vi "Main-top_feature - txtPath.vi"() -> ()   [LabVIEW 2015]
uses:
  <vilib>/Utility/file.llb/Read Delimited Spreadsheet (string).vi
  <vilib>/Utility/file.llb/Write Delimited Spreadsheet (string).vi
  <vilib>/vision/NI_Vision_Development_Module.lvlib
  EG.dll
  greenDet.dll
panel:
  out "Flower":T1(plugin-control)
  out "element":string
  in  "Date Path":path=path "H:/2-top_features_oilseed/date -whole.txt"
  in  "Save Base Path":path=path "H:/2-top_features_oilseed"
  out "交集图":T1(plugin-control)
  out "交集像素个数":dbl
  in  "Pixel Measurements 2":T2[](array[typedef])=[35] items=["Center of Mass X", "Center of Mass Y", "First Pixel X", "First Pixel Y", "Bounding Rect Left", "Bounding Rect Top", "Bounding Rect Right", "Bounding Rect Bottom", "Max Feret Diameter Start X", "Max Feret Diameter Start Y", "Max Feret Diameter End X", "Max Feret Diameter End Y", "Max Horiz. Segment Length Left", "Max Horiz. Segment Length Right", "Max Horiz. Segment Length Row", "-", "Bounding Rect Width", "Bounding Rect Height", "Bounding Rect Diagonal", "Perimeter", "Convex Hull Perimeter", "Holes' Perimeter", "Max Feret Diameter", "Equivalent Ellipse Major Axis", "Equivalent Ellipse Minor Axis", "Equivalent Ellipse Minor Axis (Feret)", "Equivalent Rect Long Side", "Equivalent Rect Short Side", "Equivalent Rect Diagonal", "Equivalent Rect Short Side (Feret)", "Average Horiz. Segment Length", "Average Vert. Segment Length", "Hydraulic Radius", "Waddel Disk Diameter", "-", "Area", "Holes' Area", "Particle & Holes' Area", "Convex Hull Area", "Image Area", "-", "Number of Holes", "Number of Horiz. Segments", "Number of Vert. Segments", "-", "Orientation", "Max Feret Diameter Orientation", "-", "% Area/Image Area", "% Area/(Particle & Holes' Area)", "Ratio of Equivalent Ellipse Axes", "Ratio of Equivalent Rect Sides", "-", "Elongation Factor", "Compactness Factor", "Heywood Circularity Factor", "Type Factor", "-", "Sum X", "Sum Y", "Sum XX", "Sum XY", "Sum YY", "Sum XXX", "Sum XXY", "Sum XYY", "Sum YYY", "-", "Moment of Inertia XX", "Moment of Inertia XY", "Moment of Inertia YY", "Moment of Inertia XXX", "Moment of Inertia XXY", "Moment of Inertia XYY", "Moment of Inertia YYY", "Norm. Moment of Inertia XX", "Norm. Moment of Inertia XY", "Norm. Moment of Inertia YY", "Norm. Moment of Inertia XXX", "Norm. Moment of Inertia XXY", "Norm. Moment of Inertia XYY", "Norm. Moment of Inertia YYY", "Hu Moment 1", "Hu Moment 2", "Hu Moment 3", "Hu Moment 4", "Hu Moment 5", "Hu Moment 6", "Hu Moment 7"]
  in  "Pixel Measurements":T2[](array[typedef])=[35] items=["Center of Mass X", "Center of Mass Y", "First Pixel X", "First Pixel Y", "Bounding Rect Left", "Bounding Rect Top", "Bounding Rect Right", "Bounding Rect Bottom", "Max Feret Diameter Start X", "Max Feret Diameter Start Y", "Max Feret Diameter End X", "Max Feret Diameter End Y", "Max Horiz. Segment Length Left", "Max Horiz. Segment Length Right", "Max Horiz. Segment Length Row", "-", "Bounding Rect Width", "Bounding Rect Height", "Bounding Rect Diagonal", "Perimeter", "Convex Hull Perimeter", "Holes' Perimeter", "Max Feret Diameter", "Equivalent Ellipse Major Axis", "Equivalent Ellipse Minor Axis", "Equivalent Ellipse Minor Axis (Feret)", "Equivalent Rect Long Side", "Equivalent Rect Short Side", "Equivalent Rect Diagonal", "Equivalent Rect Short Side (Feret)", "Average Horiz. Segment Length", "Average Vert. Segment Length", "Hydraulic Radius", "Waddel Disk Diameter", "-", "Area", "Holes' Area", "Particle & Holes' Area", "Convex Hull Area", "Image Area", "-", "Number of Holes", "Number of Horiz. Segments", "Number of Vert. Segments", "-", "Orientation", "Max Feret Diameter Orientation", "-", "% Area/Image Area", "% Area/(Particle & Holes' Area)", "Ratio of Equivalent Ellipse Axes", "Ratio of Equivalent Rect Sides", "-", "Elongation Factor", "Compactness Factor", "Heywood Circularity Factor", "Type Factor", "-", "Sum X", "Sum Y", "Sum XX", "Sum XY", "Sum YY", "Sum XXX", "Sum XXY", "Sum XYY", "Sum YYY", "-", "Moment of Inertia XX", "Moment of Inertia XY", "Moment of Inertia YY", "Moment of Inertia XXX", "Moment of Inertia XXY", "Moment of Inertia XYY", "Moment of Inertia YYY", "Norm. Moment of Inertia XX", "Norm. Moment of Inertia XY", "Norm. Moment of Inertia YY", "Norm. Moment of Inertia XXX", "Norm. Moment of Inertia XXY", "Norm. Moment of Inertia XYY", "Norm. Moment of Inertia YYY", "Hu Moment 1", "Hu Moment 2", "Hu Moment 3", "Hu Moment 4", "Hu Moment 5", "Hu Moment 6", "Hu Moment 7"]
  out "黄色分量（油菜花）二值图":T1(plugin-control)
  out "黄色分量（油菜花）":T1(plugin-control)
  out "Original Image":T1(plugin-control)
  out "Current Path":path
  out "Current Number":string
  in  "ROI_whole":T3={"Top"=550, "im_height"=1000, "L_left"=650, "im_width"=1050}
  in  "Crop image ?":bool
  out "HistStat_whole":dbl[](array[numeric])
  out "AC (Area Convexity)":dbl
  out "P":dbl
  out "TPA (Total projective area)":dbl
  out "SFD":sgl
  out "BW (minimum circumscribed box width)":dbl
  out "BH":dbl
  out "R (Rectangularity)":dbl
  out "IFD":sgl
  out "Hull area":dbl
  out "HWR":dbl
  out "greenDet":dbl
  out "Crop Image":T1(plugin-control)
  out "Final Binary Image":T1(plugin-control)
  in  "EG threshold":sgl=0.15
  in  "ER threshold":sgl=0.6
  out "Final image":T1(plugin-control)
  out "Preliminary image":T1(plugin-control)
  out "GPA (Green projective area)":dbl
  out "YPA (Yellow projective area)":dbl
  out "Image Path":path
  # "Digital evaluation software for oilseed rape phenotype-related traits (top-view) v1.0"
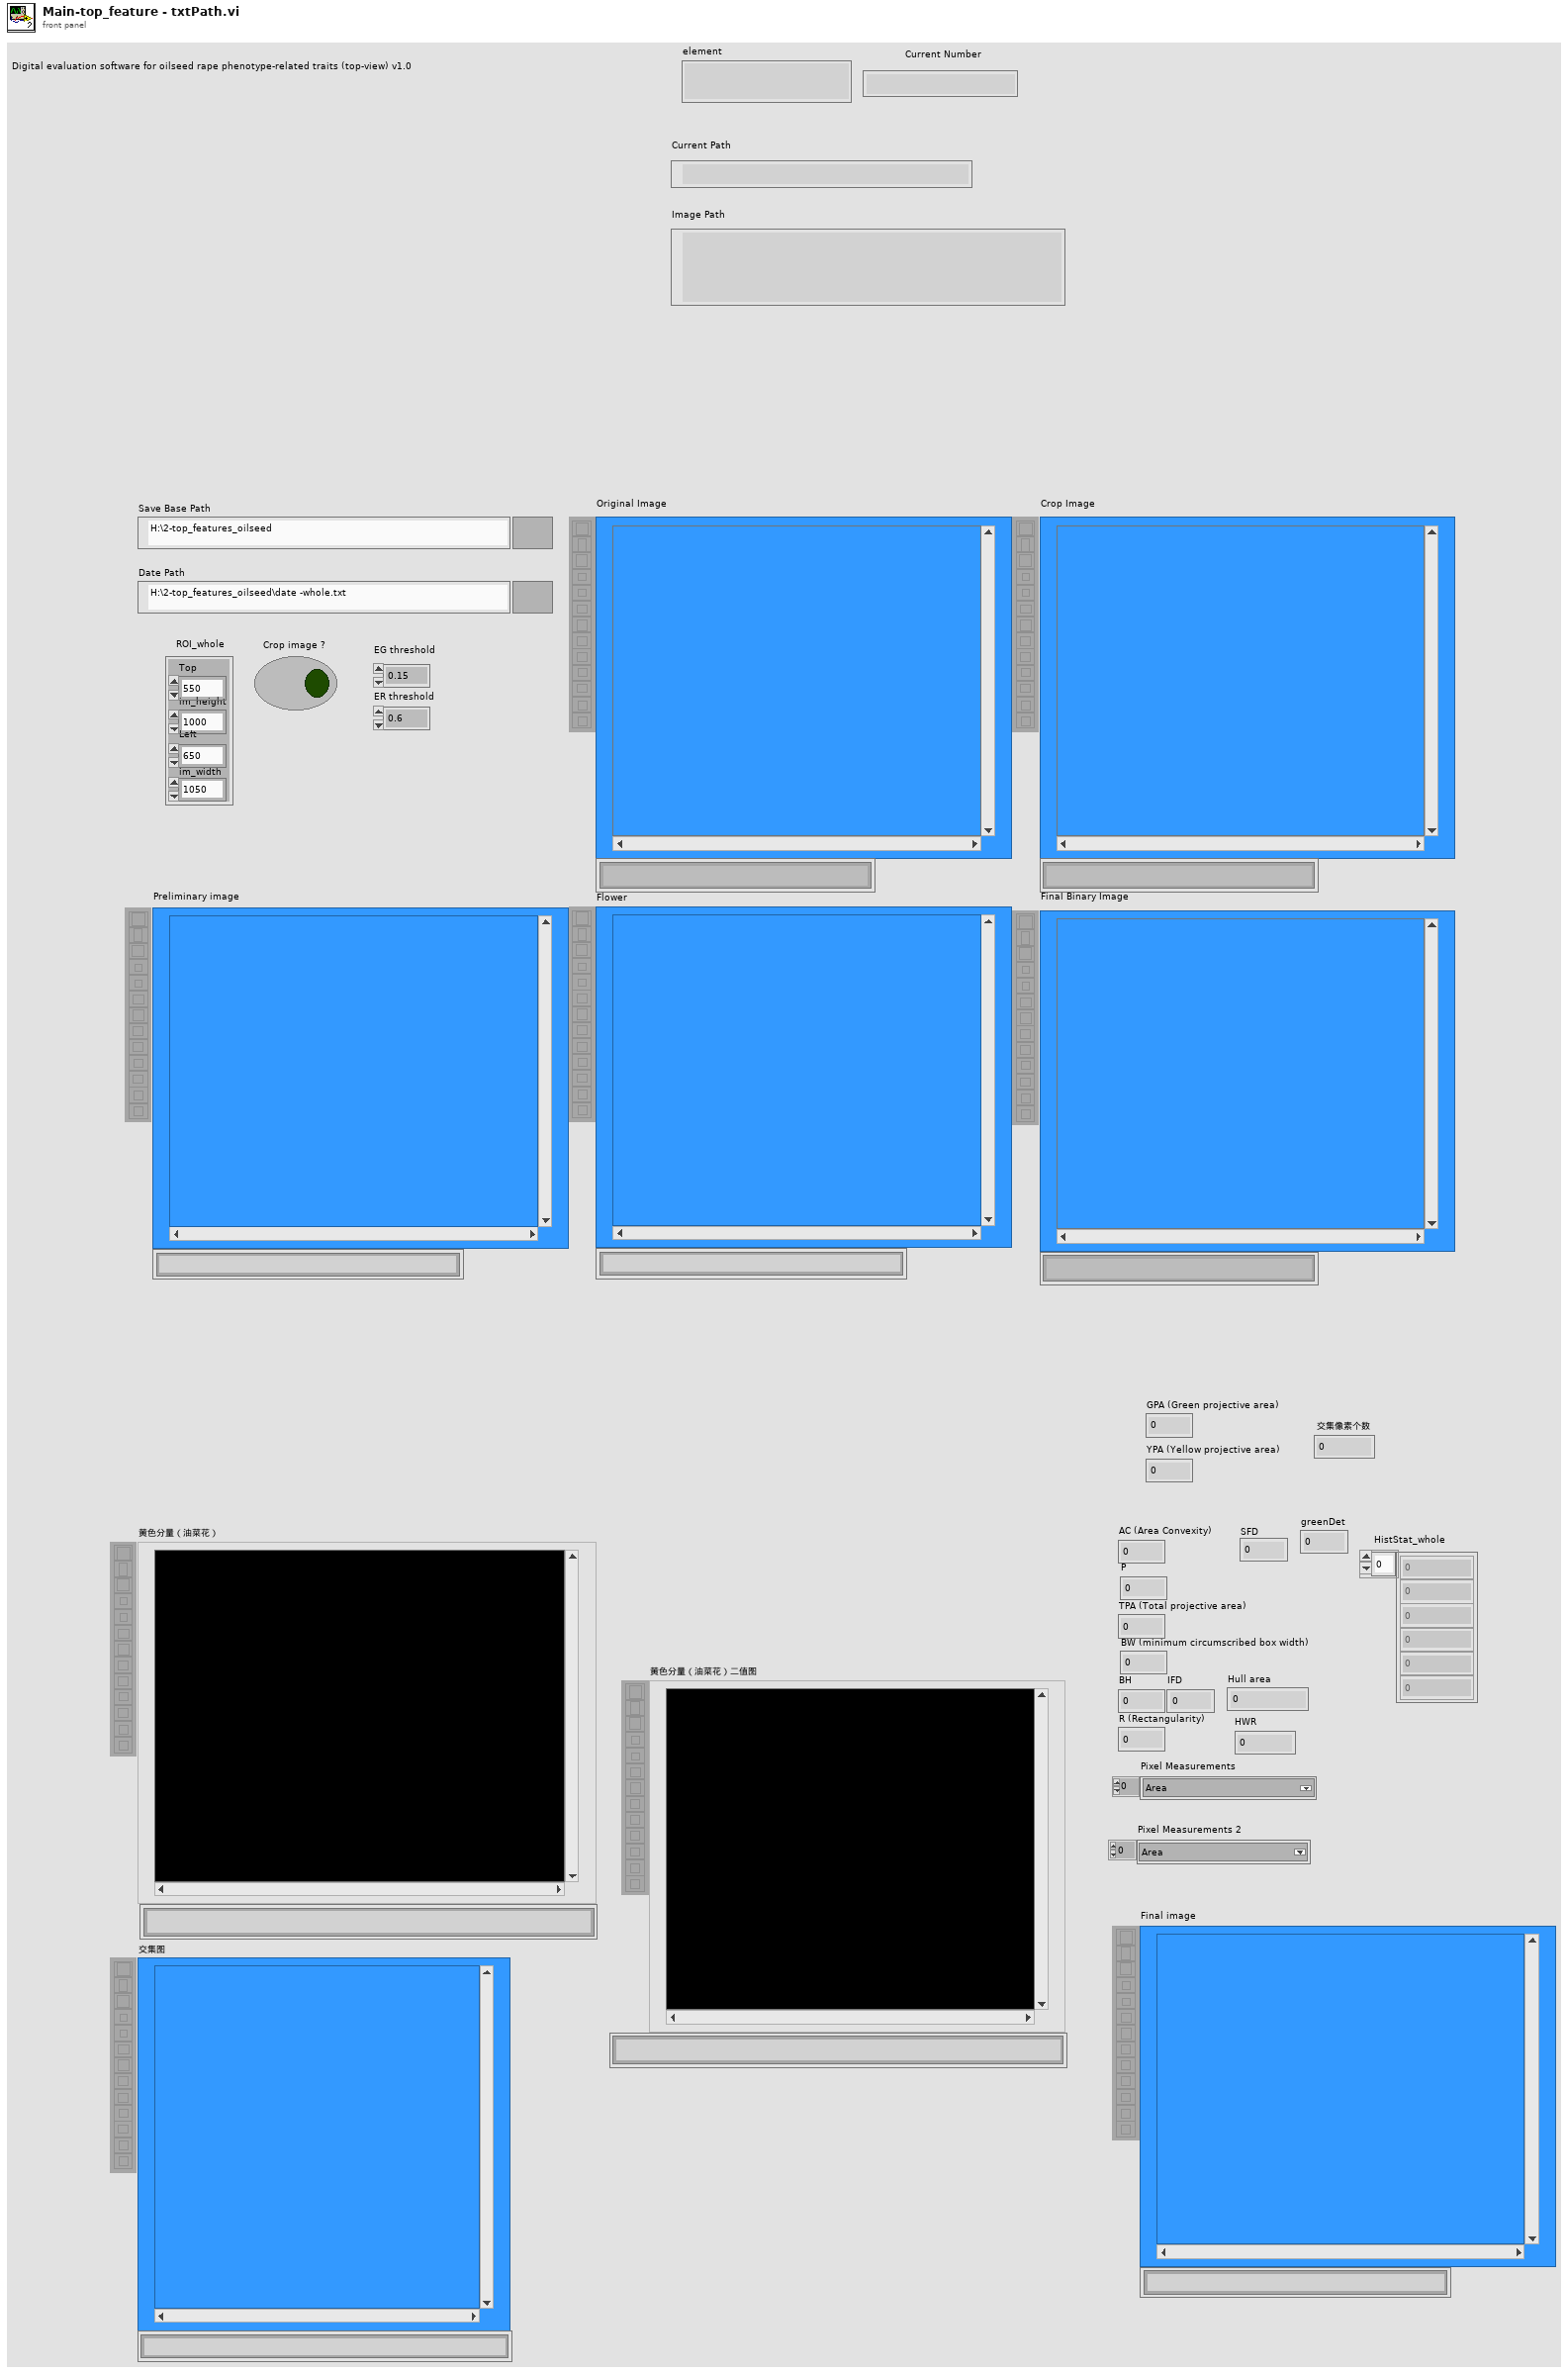
[diagram p1: front panel]
types:
  T1 = typedef "IMAQ Image.ctl" = refnum<image>
  T2 = typedef "Particle Parameters" = i32
  T3 = cluster{"Top":i32, "im_height":i32, "L_left":i32, "im_width":i32}
  T4 = enum32{"AutoM", "Close", "Dilate", "Erode", "Gradient", "Gradient out", "Gradient in", "Hit miss", "Open", "PClose", "POpen", "Thick", "Thin"}
  T5 = typedef "Image Type" = u32
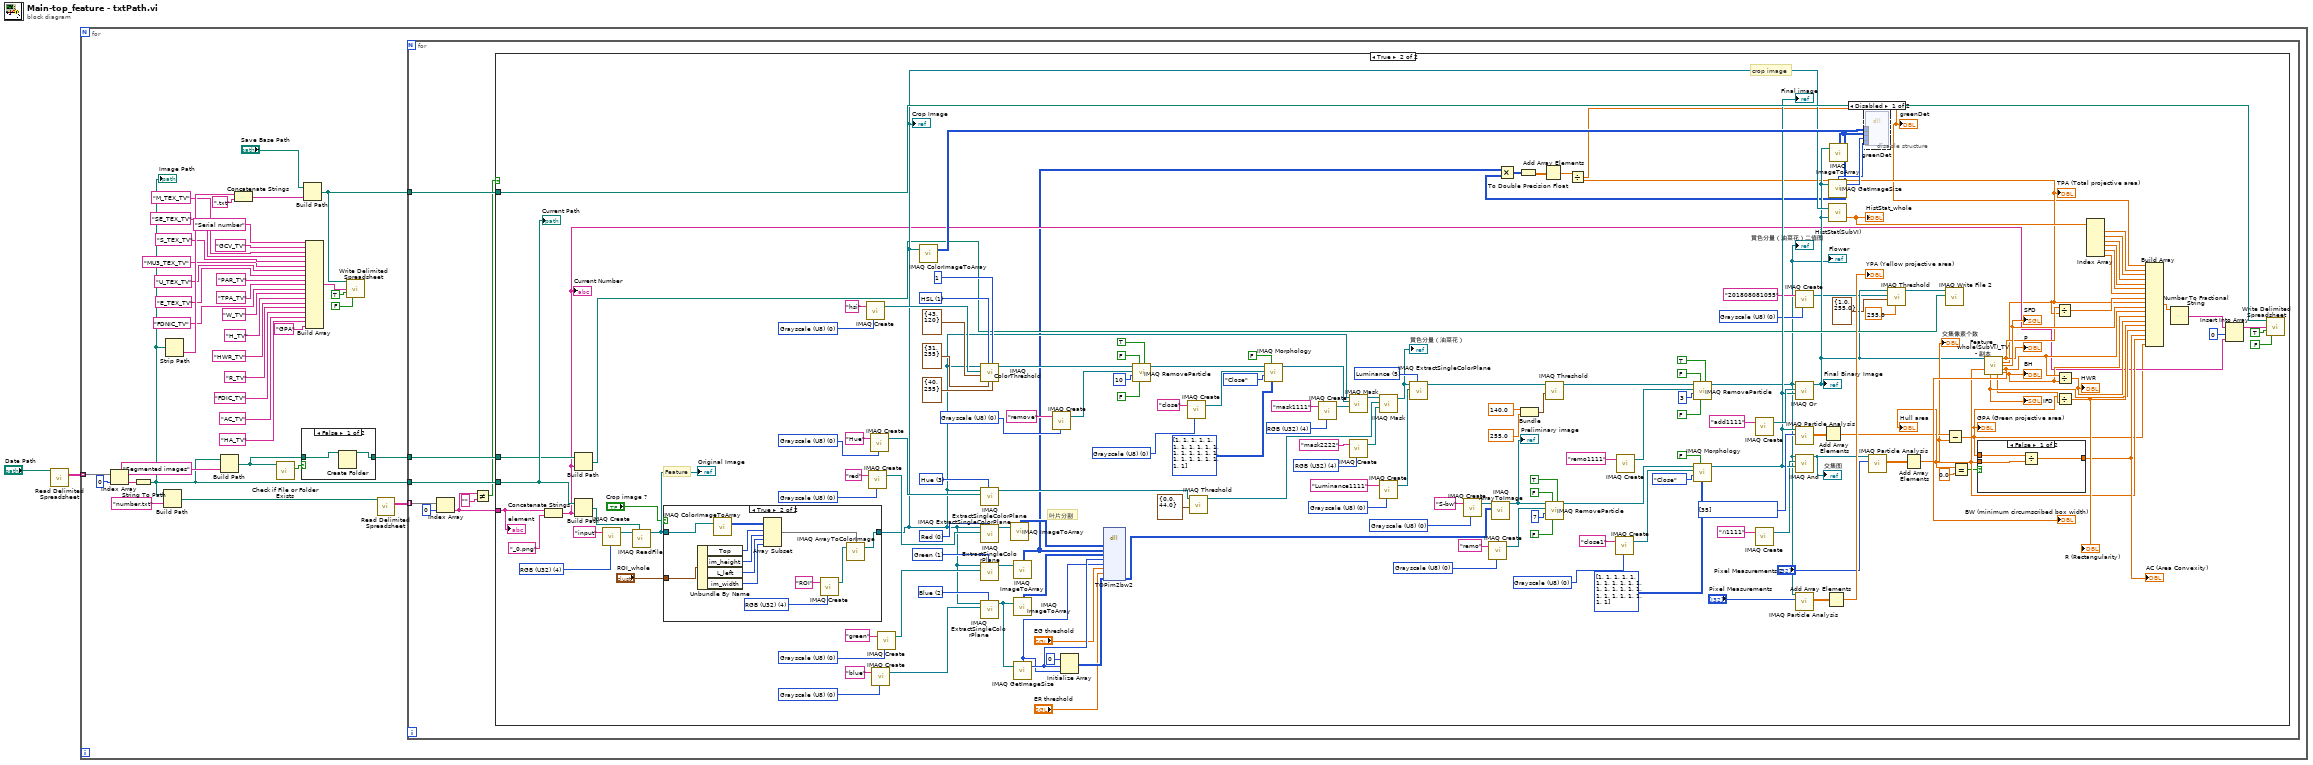
[diagram p0: block diagram]
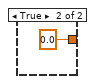
[diagram p5: hidden frame]
diagram:
  n1 = call-poly <vilib>:"Read Delimited Spreadsheet.vi"("file path (dialog if empty)"="Date Path") -> ("all rows"=w1:string[][])  [unwired: 9 in, 5 out]
  n2 = for {
    tunnel: w1 -> [w39] mode=indexing
    n3 = Index Array(array=w39, index=0) -> (element=w28:string)
    n4 = String To Path(string=w28) -> (path=w26:path)
    "Image Path" <- w26
    n5 = Build Path(base path=w26, name or relative path="number.txt") -> (appended path=w37:path)
    n6 = Strip Path(path=w26) -> (name=w27:string)  [unwired: 1 out]
    n7 = Build Path(base path=w26, name or relative path="Segmented images") -> (appended path=w33:path)
    n8 = Concatenate Strings(w27, ".txt" ("string")) -> (w30:string)
    n9 = call <vilib>:"Check if File or Folder Exists.vi"("path"=w33) -> ("file or folder exists?"=w34:bool)  [unwired: 8 in, 2 out]
    n10 = case shown="False" w34 {
      tunnel: [w41 w43] -> w32
      tunnel: w33 -> [w42 w43]
      frame False {
        n11 = Create Folder(path (use dialog)=w42) -> (created path=w41:path)  [unwired: 2 in, 2 out]
      }
      frame True {
      }
    }
    n12 = Build Path(base path="Save Base Path", name or relative path=w30) -> (appended path=w23:path)
    n13 = Build Array("Serial number" ("name or relative path"), "GCV_TV" ("name or relative path"), "M_TEX_TV" ("name or relative path"), "SE_TEX_TV" ("name or relative path"), "S_TEX_TV" ("name or relative path"), "MU3_TEX_TV" ("name or relative path"), "U_TEX_TV" ("name or relative path"), "E_TEX_TV" ("name or relative path"), "PAR_TV" ("name or relative path"), "TPA_TV" ("name or relative path"), "FDNIC_TV" ("name or relative path"), "W_TV" ("name or relative path"), "H_TV" ("name or relative path"), "HWR_TV" ("name or relative path"), "R_TV" ("name or relative path"), "FDIC_TV" ("name or relative path"), "AC_TV" ("name or relative path"), "HA_TV" ("name or relative path"), "GPA" ("name or relative path")) -> (w3:string[])
    n14 = call-poly <vilib>:"Write Delimited Spreadsheet.vi"("file path (dialog if empty)"=w23, "1D data"=w3, "append to file? (F)"=TRUE, "transpose? (F)"=FALSE ("append to file? (new file:F)")) -> ()  [unwired: 10 in, 2 out]
    n15 = call-poly <vilib>:"Read Delimited Spreadsheet.vi"("file path (dialog if empty)"=w37) -> ("all rows"=w36:string[][])  [unwired: 9 in, 5 out]
    n16 = for {
      tunnel: w26 -> [w49]
      tunnel: w36 -> [w50] mode=indexing
      tunnel: w32 -> [w48]
      tunnel: w23 -> [w47]
      n17 = Index Array(array=w50, index=0) -> (element=w46:string)
      n18 = Not Equal?(x=w46, y="") -> (x != y?=w44:bool)
      n19 = case shown="True" w44 {
        tunnel: w49 -> [_ w222]
        tunnel: w48 -> [_ w203]
        tunnel: w47 -> [_ w202]
        tunnel: w46 -> [_ w63]
        frame False {
        }
        frame True {
          w73 = u32 0 items=["Grayscale (U8)", "Grayscale (I16)", "Grayscale (SGL)", "Complex (CSG)", "RGB (U32)", "HSL (U32)", "RGB (U64)"] ("Image Type")
          w102 = u32 0 items=["Grayscale (U8)", "Grayscale (I16)", "Grayscale (SGL)", "Complex (CSG)", "RGB (U32)", "HSL (U32)", "RGB (U64)"] ("Image Type")
          w105 = 5 items=["Red", "Green", "Blue", "Hue", "Saturation", "Luminance", "Value", "Intensity"] ("Color Plane")
          w109 = u32 0 items=["Grayscale (U8)", "Grayscale (I16)", "Grayscale (SGL)", "Complex (CSG)", "RGB (U32)", "HSL (U32)", "RGB (U64)"] ("Image Type")
          w112 = 3 items=["Red", "Green", "Blue", "Hue", "Saturation", "Luminance", "Value", "Intensity"] ("Color Plane")
          w115 = u32 4 items=["Grayscale (U8)", "Grayscale (I16)", "Grayscale (SGL)", "Complex (CSG)", "RGB (U32)", "HSL (U32)", "RGB (U64)"] ("Image Type")
          w118 = u32 4 items=["Grayscale (U8)", "Grayscale (I16)", "Grayscale (SGL)", "Complex (CSG)", "RGB (U32)", "HSL (U32)", "RGB (U64)"] ("Image Type")
          w127 = u32 0 items=["Grayscale (U8)", "Grayscale (I16)", "Grayscale (SGL)", "Complex (CSG)", "RGB (U32)", "HSL (U32)", "RGB (U64)"] ("Image Type")
          w131 = T2[] [35] items=["Center of Mass X", "Center of Mass Y", "First Pixel X", "First Pixel Y", "Bounding Rect Left", "Bounding Rect Top", "Bounding Rect Right", "Bounding Rect Bottom", "Max Feret Diameter Start X", "Max Feret Diameter Start Y", "Max Feret Diameter End X", "Max Feret Diameter End Y", "Max Horiz. Segment Length Left", "Max Horiz. Segment Length Right", "Max Horiz. Segment Length Row", "-", "Bounding Rect Width", "Bounding Rect Height", "Bounding Rect Diagonal", "Perimeter", "Convex Hull Perimeter", "Holes' Perimeter", "Max Feret Diameter", "Equivalent Ellipse Major Axis", "Equivalent Ellipse Minor Axis", "Equivalent Ellipse Minor Axis (Feret)", "Equivalent Rect Long Side", "Equivalent Rect Short Side", "Equivalent Rect Diagonal", "Equivalent Rect Short Side (Feret)", "Average Horiz. Segment Length", "Average Vert. Segment Length", "Hydraulic Radius", "Waddel Disk Diameter", "-", "Area", "Holes' Area", "Particle & Holes' Area", "Convex Hull Area", "Image Area", "-", "Number of Holes", "Number of Horiz. Segments", "Number of Vert. Segments", "-", "Orientation", "Max Feret Diameter Orientation", "-", "% Area/Image Area", "% Area/(Particle & Holes' Area)", "Ratio of Equivalent Ellipse Axes", "Ratio of Equivalent Rect Sides", "-", "Elongation Factor", "Compactness Factor", "Heywood Circularity Factor", "Type Factor", "-", "Sum X", "Sum Y", "Sum XX", "Sum XY", "Sum YY", "Sum XXX", "Sum XXY", "Sum XYY", "Sum YYY", "-", "Moment of Inertia XX", "Moment of Inertia XY", "Moment of Inertia YY", "Moment of Inertia XXX", "Moment of Inertia XXY", "Moment of Inertia XYY", "Moment of Inertia YYY", "Norm. Moment of Inertia XX", "Norm. Moment of Inertia XY", "Norm. Moment of Inertia YY", "Norm. Moment of Inertia XXX", "Norm. Moment of Inertia XXY", "Norm. Moment of Inertia XYY", "Norm. Moment of Inertia YYY", "Hu Moment 1", "Hu Moment 2", "Hu Moment 3", "Hu Moment 4", "Hu Moment 5", "Hu Moment 6", "Hu Moment 7"] ("Pixel Measurements")
          w164 = T5 0 items=["Grayscale (U8)", "Grayscale (I16)", "Grayscale (SGL)", "Complex (CSG)", "RGB (U32)", "HSL (U32)", "RGB (U64)", "Grayscale (U16)"] ("Image Type")
          w157 = T5 0 items=["Grayscale (U8)", "Grayscale (I16)", "Grayscale (SGL)", "Complex (CSG)", "RGB (U32)", "HSL (U32)", "RGB (U64)", "Grayscale (U16)"] ("Image Type")
          w144 = 2 items=["Red", "Green", "Blue", "Hue", "Saturation", "Luminance", "Value", "Intensity"] ("Color Plane")
          w143 = 0 items=["Red", "Green", "Blue", "Hue", "Saturation", "Luminance", "Value", "Intensity"] ("Color Plane")
          w140 = T5 0 items=["Grayscale (U8)", "Grayscale (I16)", "Grayscale (SGL)", "Complex (CSG)", "RGB (U32)", "HSL (U32)", "RGB (U64)", "Grayscale (U16)"] ("Image Type")
          w138 = 1 items=["Red", "Green", "Blue", "Hue", "Saturation", "Luminance", "Value", "Intensity"] ("Color Plane")
          w135 = T5 0 items=["Grayscale (U8)", "Grayscale (I16)", "Grayscale (SGL)", "Complex (CSG)", "RGB (U32)", "HSL (U32)", "RGB (U64)", "Grayscale (U16)"] ("Image Type")
          w139 = T5 0 items=["Grayscale (U8)", "Grayscale (I16)", "Grayscale (SGL)", "Complex (CSG)", "RGB (U32)", "HSL (U32)", "RGB (U64)", "Grayscale (U16)"] ("Image Type")
          w168 = u32 0 items=["Grayscale (U8)", "Grayscale (I16)", "Grayscale (SGL)", "Complex (CSG)", "RGB (U32)", "HSL (U32)", "RGB (U64)"] ("Image Type")
          w179 = u32 0 items=["Grayscale (U8)", "Grayscale (I16)", "Grayscale (SGL)", "Complex (CSG)", "RGB (U32)", "HSL (U32)", "RGB (U64)"] ("Image Type")
          w182 = u32 0 items=["Grayscale (U8)", "Grayscale (I16)", "Grayscale (SGL)", "Complex (CSG)", "RGB (U32)", "HSL (U32)", "RGB (U64)"] ("Image Type")
          w184 = u16 1 items=["RGB", "HSL", "HSV", "HSI"] ("Color Mode")
          w199 = T5 4 items=["Grayscale (U8)", "Grayscale (I16)", "Grayscale (SGL)", "Complex (CSG)", "RGB (U32)", "HSL (U32)", "RGB (U64)", "Grayscale (U16)"] ("Image Type")
          # "叶片分割"
          # "crop image"
          # "Feature"
          n20 = Concatenate Strings(w63, "_0.png" ("string")) -> (w61:string)
          "Current Number" <- w61
          n21 = Build Path(base path=w203, name or relative path=w61) -> (appended path=w75:path)
          n22 = Build Path(base path=w222, name or relative path=w61) -> (appended path=w198:path)
          n23 = call "IMAQ Create"("Image Name"="input", "Image Type"=w199) -> ("New Image"=w200:T1)  [unwired: 2 in, 2 out]
          n24 = call "IMAQ ReadFile"("File Path"=w198, "Image"=w200) -> ("Image Out"=w196:T1)  [unwired: 3 in, 6 out]
          "Original Image" <- w196
          n25 = case shown="True" "Crop image ?" {
            tunnel: w196 -> [w231 w238]
            tunnel: "ROI_whole" -> [_ w233]
            tunnel: [w231 w232] -> w87
            frame False {
            }
            frame True {
              w236 = u32 4 items=["Grayscale (U8)", "Grayscale (I16)", "Grayscale (SGL)", "Complex (CSG)", "RGB (U32)", "HSL (U32)", "RGB (U64)"] ("Image Type")
              n26 = Unbundle By Name(w233) -> ("Top"=w240:i32, "im_height"=w241:i32, "L_left"=w242:i32, "im_width"=w243:i32)
              n27 = call "IMAQ ColorImageToArray"("Image"=w238) -> ("Image Pixels (U32)"=w239:u32[][])  [unwired: 2 in, 3 out]
              n28 = Array Subset(array=w239, index (row)=w240, length (row)=w241, index (col)=w242, length (col)=w243) -> (w234:u32[][])
              n29 = call "IMAQ Create"("Image Name"="ROI", "Image Type"=w236) -> ("New Image"=w235:T1)  [unwired: 2 in, 2 out]
              n30 = call "IMAQ ArrayToColorImage"("Image Pixels (U32)"=w234, "Image"=w235) -> ("Image Out"=w232:T1)  [unwired: 2 in, 2 out]
            }
          }
          "Crop Image" <- w87
          n31 = call "IMAQ Create"("Image Name"="hsi", "Image Type"=w182) -> ("New Image"=w181:T1)  [unwired: 2 in, 2 out]
          n32 = call "IMAQ Create"("Image Name"="red", "Image Type"=w139) -> ("New Image"=w134:T1)  [unwired: 2 in, 2 out]
          n33 = call "IMAQ Create"("Image Name"="Hue", "Image Type"=w109) -> ("New Image"=w108:T1)  [unwired: 2 in, 2 out]
          n34 = call "IMAQ Create"("Image Name"="blue", "Image Type"=w135) -> ("New Image"=w137:T1)  [unwired: 2 in, 2 out]
          n35 = call "IMAQ Create"("Image Name"="green", "Image Type"=w140) -> ("New Image"=w142:T1)  [unwired: 2 in, 2 out]
          n36 = call "IMAQ ColorImageToArray"("Image"=w87) -> ("Image Pixels (U32)"=w177:u32[][])  [unwired: 2 in, 3 out]
          n37 = call "IMAQ ColorThreshold"("Blue or Luma or Val or Inten Range"=cluster{"Lower value":i32, "Upper value":i32} {"Lower value"=40, "Upper value"=255}, "Replace Value"=1, "Green or Sat Range"=cluster{"Lower value":i32, "Upper value":i32} {"Lower value"=31, "Upper value"=255}, "Color Mode"=w184, "Red or Hue Range"=cluster{"Lower value":i32, "Upper value":i32} {"Lower value"=43, "Upper value"=120}, "Image Dst"=w181, "Image Src"=w87) -> ("Image Dst Out"=w185:T1)  [unwired: 1 in, 3 out]
          n38 = call "IMAQ ExtractSingleColorPlane"("Color Plane"=w112, "Image Dst"=w108, "Image Src"=w87) -> ("Image Dst Out"=w110:T1)  [unwired: 1 in, 7 out]
          n39 = call "IMAQ ExtractSingleColorPlane"("Color Plane"=w143, "Image Dst"=w134, "Image Src"=w87) -> ("Image Dst Out"=w146:T1)  [unwired: 1 in, 7 out]
          n40 = call "IMAQ ExtractSingleColorPlane"("Color Plane"=w138, "Image Dst"=w142, "Image Src"=w87) -> ("Image Dst Out"=w145:T1)  [unwired: 1 in, 7 out]
          n41 = call "IMAQ ExtractSingleColorPlane"("Color Plane"=w144, "Image Dst"=w137, "Image Src"=w87) -> ("Image Dst Out"=w149:T1)  [unwired: 1 in, 7 out]
          n42 = call "IMAQ ImageToArray"("Image"=w146) -> ("Image Pixels (U8)"=w147:u8[][])  [unwired: 2 in, 5 out]
          n43 = call "IMAQ ImageToArray"("Image"=w145) -> ("Image Pixels (U8)"=w59:u8[][])  [unwired: 2 in, 5 out]
          n44 = call "IMAQ ImageToArray"("Image"=w149) -> ("Image Pixels (U8)"=w148:u8[][])  [unwired: 2 in, 5 out]
          n45 = call "IMAQ GetImageSize"("Image"=w149) -> ("Y Resolution"=w154:i32, "X Resolution"=w153:i32)  [unwired: 1 in, 3 out]
          n46 = call "IMAQ Create"("Image Name"="remove", "Image Type"=w179) -> ("New Image"=w178:T1)  [unwired: 2 in, 2 out]
          n47 = Initialize Array(u8 0 ("element"), w154, w153) -> (w155:u8[][])
          n48 = dll-call lib="H:/2-top_features_oilseed/EG.dll" fn="TOPim2bw2"("R"=w147, "G"=w59, "B"=w148, "row"=w154, "col"=w153, "EGthreshold"="EG threshold", "ERthreshold"="ER threshold", "bw"=w155) -> ("bw"=w159:u8[][])  [unwired: 10 in, 3 out]
          n49 = call "IMAQ RemoveParticle"("Connectivity 4/8 (8)"=TRUE, "Low Pass/High Pass (Low)"=FALSE, "Square/Hexa (Square)"=FALSE, "Number of Erosion"=10, "Image Dst"=w178, "Image Src"=w185) -> ("Image Dst Out"=w170:T1)  [unwired: 1 in, 4 out]
          n50 = call "IMAQ Create"("Image Name"="close", "Image Type"=w168) -> ("New Image"=w167:T1)  [unwired: 2 in, 2 out]
          n51 = call "IMAQ Threshold"("Range"=cluster{"Lower value":sgl, "Upper value":sgl} {"Lower value"=0.0, "Upper value"=44.0}, "Image Src"=w110) -> ("Image Dst Out"=w88:T1)  [unwired: 4 in, 5 out]
          n52 = call "IMAQ Morphology"("Structuring Element"=i32[][] [[1, 1, 1, 1, 1], [1, 1, 1, 1, 1], [1, 1, 1, 1, 1], [1, 1, 1, 1, 1], [1, 1, 1, 1, 1]], "Square/Hexa (Square)"=FALSE, "Operation"=T4."Close", "Image Dst"=w167, "Image Src"=w170) -> ("Image Dst Out"=w85:T1)  [unwired: 2 in, 4 out]
          n53 = call "IMAQ Create"("Image Name"="mask1111", "Image Type"=w118) -> ("New Image"=w117:T1)  [unwired: 2 in, 2 out]
          n54 = call "IMAQ Mask"("Image Dst"=w117, "Image Mask"=w85, "Image Src"=w87) -> ("Image Dst Out"=w113:T1)  [unwired: 1 in, 2 out]
          n55 = call "IMAQ Create"("Image Name"="mask2222", "Image Type"=w115) -> ("New Image"=w114:T1)  [unwired: 2 in, 2 out]
          n56 = call "IMAQ Mask"("Image Dst"=w114, "Image Mask"=w88, "Image Src"=w113) -> ("Image Dst Out"=w103:T1)  [unwired: 1 in, 2 out]
          "黄色分量（油菜花）" <- w103
          n57 = call "IMAQ Create"("Image Name"="Luminance1111", "Image Type"=w102) -> ("New Image"=w104:T1)  [unwired: 2 in, 2 out]
          n58 = call "IMAQ ExtractSingleColorPlane"("Color Plane"=w105, "Image Dst"=w104, "Image Src"=w103) -> ("Image Dst Out"=w106:T1)  [unwired: 1 in, 7 out]
          n59 = call "IMAQ Create"("Image Name"="S-bw", "Image Type"=w157) -> ("New Image"=w158:T1)  [unwired: 2 in, 2 out]
          n60 = call "IMAQ Create"("Image Name"="remo", "Image Type"=w164) -> ("New Image"=w166:T1)  [unwired: 2 in, 2 out]
          n61 = call "IMAQ ArrayToImage"("Image Pixels (U8)"=w159, "Image"=w158) -> ("Image Out"=w124:T1)  [unwired: 4 in, 5 out]
          "Preliminary image" <- w124
          n62 = Bundle("Lower value"=sgl 140.0, "Upper value"=sgl 255.0) -> (w98:cluster{"Lower value":sgl, "Upper value":sgl})  [unwired: 1 in]
          n63 = call "IMAQ Threshold"("Range"=w98, "Image Src"=w106) -> ("Image Dst Out"=w90:T1)  [unwired: 4 in, 5 out]
          n64 = call "IMAQ RemoveParticle"("Connectivity 4/8 (8)"=TRUE, "Low Pass/High Pass (Low)"=FALSE, "Square/Hexa (Square)"=FALSE, "Number of Erosion"=7, "Image Dst"=w166, "Image Src"=w124) -> ("Image Dst Out"=w123:T1)  [unwired: 1 in, 4 out]
          n65 = call "IMAQ Create"("Image Name"="close1", "Image Type"=w127) -> ("New Image"=w126:T1)  [unwired: 2 in, 2 out]
          n66 = call "IMAQ Create"("Image Name"="remo1111") -> ("New Image"=w91:T1)  [unwired: 3 in, 2 out]
          n67 = call "IMAQ RemoveParticle"("Connectivity 4/8 (8)"=TRUE, "Low Pass/High Pass (Low)"=FALSE, "Square/Hexa (Square)"=FALSE, "Number of Erosion"=3, "Image Dst"=w91, "Image Src"=w90) -> ("Image Dst Out"=w52:T1)  [unwired: 1 in, 4 out]
          "黄色分量（油菜花）二值图" <- w52
          "Flower" <- w52
          n68 = call "IMAQ Morphology"("Structuring Element"=i32[][] [[1, 1, 1, 1, 1], [1, 1, 1, 1, 1], [1, 1, 1, 1, 1], [1, 1, 1, 1, 1], [1, 1, 1, 1, 1]], "Square/Hexa (Square)"=FALSE, "Operation"=T4."Close", "Image Dst"=w126, "Image Src"=w123) -> ("Image Dst Out"=w83:T1)  [unwired: 2 in, 4 out]
          "Final image" <- w83
          n69 = call "IMAQ Create"("Image Name"="add1111") -> ("New Image"=w84:T1)  [unwired: 3 in, 2 out]
          n70 = call "IMAQ Create"("Image Name"="∩1111") -> ("New Image"=w81:T1)  [unwired: 3 in, 2 out]
          n71 = call "IMAQ Create"("Image Name"="201808081055", "Image Type"=w73) -> ("New Image"=w71:T1)  [unwired: 2 in, 2 out]
          n72 = call "IMAQ Or"("Image Src B"=w83, "Image Dst"=w84, "Image Src A"=w52) -> ("Image Dst Out"=w74:T1)  [unwired: 7 in, 1 out]
          "Final Binary Image" <- w74
          n73 = call "IMAQ Particle Analysis"("Pixel Measurements"=w131, "Image"=w83) -> ("Particle Measurements (Pixels)"=w132:dbl[][])  [unwired: 3 in, 6 out]
          n74 = call "IMAQ And"("Image Src B"=w83, "Image Dst"=w81, "Image Src A"=w52) -> ("Image Dst Out"=w77:T1)  [unwired: 7 in, 1 out]
          "交集图" <- w77
          n75 = call "IMAQ Particle Analysis"("Pixel Measurements"="Pixel Measurements", "Image"=w52) -> ("Particle Measurements (Pixels)"=w97:dbl[][])  [unwired: 3 in, 6 out]
          n76 = Add Array Elements(numeric array=w132) -> (sum=w78:dbl)
          n77 = Add Array Elements(numeric array=w97) -> (sum=→"YPA (Yellow projective area)":dbl)
          n78 = call "IMAQ GetImageSize"("Image"=w74) -> ("Y Resolution"=w176:i32, "X Resolution"=w175:i32)  [unwired: 1 in, 3 out]
          n79 = call "HistStat(SubVI).vi"("Binary Image"=w74, "Original Image"=w87) -> ("HistStat"=w174:dbl[])  [unwired: 1 out]
          "HistStat_whole" <- w174
          n80 = call "IMAQ ImageToArray"("Image"=w74) -> ("Image Pixels (U8)"=w58:u8[][])  [unwired: 2 in, 5 out]
          n81 = Multiply(x=w59, y=w58) -> (x*y=w57:u8[][])
          n82 = To Double Precision Float(number=w57) -> (double precision float=w56:dbl[][])
          n83 = Add Array Elements(numeric array=w56) -> (sum=w55:dbl)
          n84 = disable-structure shown="Disabled" {
            disable-tunnel: w177 -> [w226 _]
            disable-tunnel: w176 -> [w225 _]
            disable-tunnel: w175 -> [w224 _]
            disable-tunnel: w58 -> [w223 _]
            frame Disabled {
              n85 = dll-call lib="H:/2-top_features_oilseed/greenDet.dll" fn="greenDet"("oriArray"=w226, "binArray"=w223, "imageRows"=w225, "imageCols"=w224) -> ()  [unwired: 7 in, 3 out]
            }
            frame Enabled {
            }
          }
          n86 = call "IMAQ Particle Analysis"("Pixel Measurements"="Pixel Measurements 2", "Image"=w77) -> ("Particle Measurements (Pixels)"=w80:dbl[][])  [unwired: 3 in, 6 out]
          n87 = call "IMAQ Threshold"("Replace Value"=sgl 255.0, "Range"=cluster{"Lower value":sgl, "Upper value":sgl} {"Lower value"=1.0, "Upper value"=255.0}, "Image Dst"=w71, "Image Src"=w74) -> ("Image Dst Out"=w68:T1)  [unwired: 6 in, 1 out]
          n88 = Add Array Elements(numeric array=w80) -> (sum=w76:dbl)
          "交集像素个数" <- w76
          n89 = call-poly "IMAQ Write File 2"("File Path"=w75, "Image"=w68) -> ()  [unwired: 8 in, 2 out]
          n90 = Subtract(x=w78, y=w76) -> (x-y=w60:dbl)
          "GPA (Green projective area)" <- w60
          n91 = call "Feature_whole(SubVI)_TV - 副本.vi"("Binary Image"=w74) -> ("P"=w204:dbl, "SA"=w54:dbl, "SFD"=w220:sgl, "Hull area"=w213:dbl, "SW"=w219:dbl, "IFD"=w215:sgl, "最小外接矩面积"=w122:dbl, "SH"=w218:dbl)  [unwired: 6 in, 1 out]
          "P" <- w204
          "TPA (Total projective area)" <- w54
          "SFD" <- w220
          "BW (minimum circumscribed box width)" <- w219
          "BH" <- w218
          "IFD" <- w215
          "Hull area" <- w213
          n92 = Divide(x=w55, y=w54) -> (x/y=w53:dbl)
          "greenDet" <- w53
          n93 = Equal?(x=w213, y=0.0) -> (x = y?=w121:bool)
          n94 = case shown="False" w121 {
            tunnel: w60 -> [w229 _]
            tunnel: w213 -> [w228 _]
            tunnel: [w227 0.0] -> w214
            frame False {
              n95 = Divide(x=w229, y=w228) -> (x/y=w227:dbl)
            }
            frame True {
            }
          }
          "AC (Area Convexity)" <- w214
          n96 = Divide(x=w204, y=w54) -> (x/y=w221:dbl)
          n97 = Divide(x=w219, y=w218) -> (x/y=w217:dbl)
          "HWR" <- w217
          n98 = Divide(x=w60, y=w122) -> (x/y=w216:dbl)
          "R (Rectangularity)" <- w216
          n99 = Index Array(array=w174) -> (element #1=w212:dbl, element #2=w211:dbl, element #3=w210:dbl, element #4=w209:dbl, element #5=w208:dbl, element #6=w207:dbl)  [unwired: 6 in]
          n100 = Build Array(w53, w212, w211, w210, w209, w208, w207, w221, w54, w220, w219, w218, w217, w216, w215, w214, w213, w60) -> (w66:dbl[])
          n101 = Number To Fractional String(number=w66) -> (F-format string=w65:string[])  [unwired: 3 in]
          n102 = Insert Into Array(array=w65, index=0, new element=w61) -> (w62:string[])
          n103 = call-poly <vilib>:"Write Delimited Spreadsheet.vi"("file path (dialog if empty)"=w202, "1D data"=w62, "append to file? (F)"=TRUE, "transpose? (F)"=FALSE ("append to file? (new file:F)")) -> ()  [unwired: 10 in, 2 out]
          "Current Path" <- w222
          "element" <- w63
        }
      }
    }
  }
